vi "testFlattenTimeToXML.vi"() -> ()   [LabVIEW 2012, in "UnitsAndXML.lvlib"]
uses:
  <userlib>/Common/UnitsAndXML/UnitsAndXML.lvlib
  <userlib>/Common/UnitsAndXML/FlattenItemWithUnitToXML/FlattenTimeToXML/TimeUnit.ctl
  <userlib>/Common/UnitsAndXML/FlattenItemWithUnitToXML/FlattenTimeToXML/typeMethods/flattenTimeToXML_Array.vi
  <userlib>/Common/UnitsAndXML/FlattenItemWithUnitToXML/FlattenTimeToXML/typeMethods/flattenTimeToXML_Scalar.vi
panel:
  out "error out":errorcluster
  in  "timeUnitInXML":T1
  out "xmlStringArray":string
  out "xmlStringScalar":string
  in  "time":dbl[unit][](array[numeric])=[899.9999999999999, 1799.9999999999998, 2700.0, 3599.9999999999995]
  in  "time":dbl[unit]=899.9999999999999
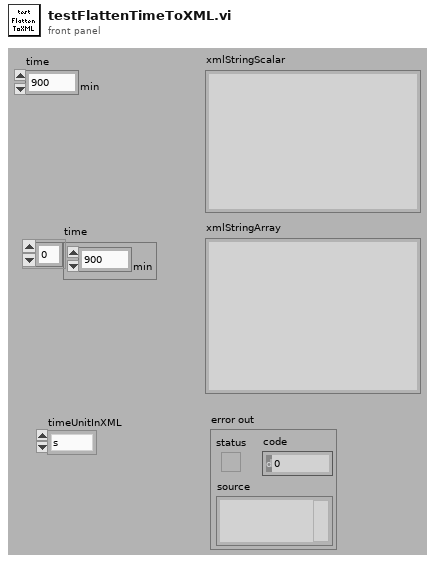
[diagram p1: front panel]
types:
  T1 = typedef "UnitsAndXML.lvlib/TimeUnit.ctl" = enum16{"s", "d", "h", "min", "a"}
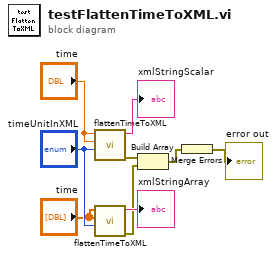
[diagram p0: block diagram]
diagram:
  n1 = call-poly <userlib>:"flattenTimeToXML.vi"("timeUnitInXML"="timeUnitInXML", "timeAgain"="time", "time"="time") -> ("error out"=w6:errorcluster, "xmlString"=→"xmlStringScalar":string)  [unwired: 7 in]
  n2 = call-poly <userlib>:"flattenTimeToXML.vi"("timeUnitInXML"="timeUnitInXML", "timeAgain"="time", "time"="time") -> ("error out"=w1:errorcluster, "xmlString"=→"xmlStringArray":string)  [unwired: 7 in]
  n3 = Build Array(w6, w1) -> (w7:errorcluster[])
  n4 = Merge Errors(w7) -> (→"error out":errorcluster)
